vi "Write State to Bus.vi"(8 "error in (no error)":errorcluster, 10 "Channel":T1, 11 "MCP23017 in":refnum<class "MCP23017.lvclass">) -> (0 "error out":errorcluster, 3 "MCP23017 out":refnum<class "MCP23017.lvclass">)   [LabVIEW 2020, in "MCP23017.lvclass"]
uses:
  MCP23017.lvclass
  MCP23017.lvclass/MCP23017.ctl
  GPIO Channel.ctl
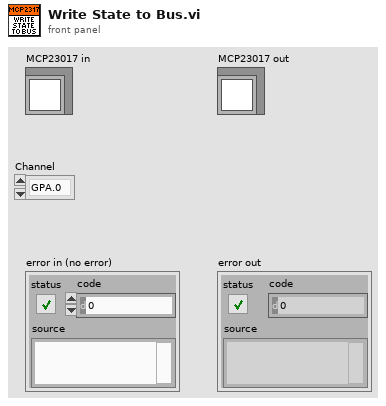
[diagram p1: front panel]
types:
  T1 = typedef "GPIO Channel.ctl" = enum16{"GPA.0", "GPA.1", "GPA.2", "GPA.3", "GPA.4", "GPA.5", "GPA.6", "GPA.7", "GPB.0", "GPB.1", "GPB.2", "GPB.3", "GPB.4", "GPB.5", "GPB.6", "GPB.7"}
  T2 = typedef "MCP23017.lvclass/Registers.ctl" = u16
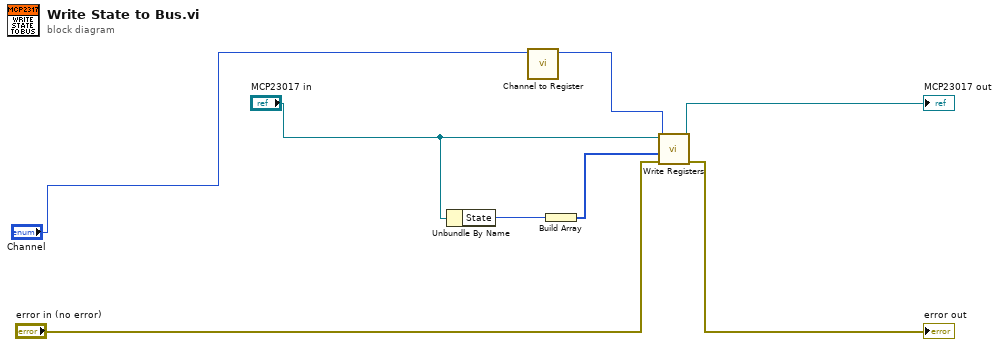
[diagram p0: block diagram]
diagram:
  n1 = Unbundle By Name("MCP23017 in") -> ("State"=w8:u8)
  n2 = call "Channel to Register.vi"("Channel"="Channel") -> ("f"=w4:T2)  [unwired: 10 in]
  n3 = Build Array(w8) -> (w6:u8[])
  n4 = call "Write Registers.vi"("error in (no error)"="error in (no error)", "Data"=w6, "Registers"=w4, "MCP23017 in"="MCP23017 in") -> ("error out"=→"error out":errorcluster, "MCP23017 out"=→"MCP23017 out":refnum<class "MCP23017.lvclass">)  [unwired: 6 in]
